vi "Flatten Value.vi"(8 "Error In":errorcluster, 11 "2D Path In":refnum<class "2D Path.lvclass">) -> (0 "Error Out":errorcluster, 1 "Value":string, 3 "2D Path Out":refnum<class "2D Path.lvclass">)   [LabVIEW 2017, in "Tree API.lvlib" / "2D Path.lvclass"]
doc: "Dynamic dispatch interface for flattening Tree Data classes to string."
uses:
  2D Path.lvclass
  Tree Manager/Tree.lvclass
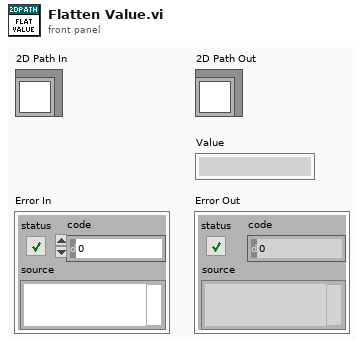
[diagram p1: front panel]
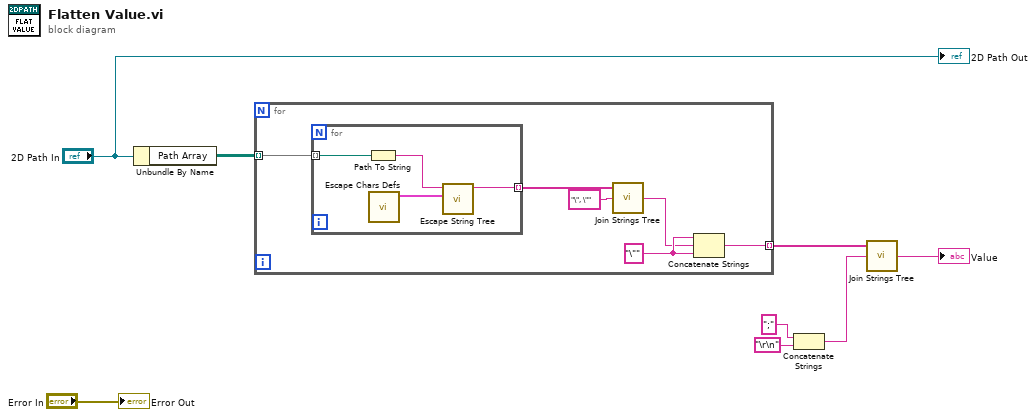
[diagram p0: block diagram]
diagram:
  n1 = Unbundle By Name("2D Path In") -> ("Path Array"=w8:path[][])
  n2 = for {
    tunnel: w8 -> [w14] mode=indexing
    tunnel: [w9] -> w6 mode=indexing
    w12 = "\"" ("string")
    n3 = for {
      tunnel: w14 -> [w18] mode=indexing
      tunnel: [w15] -> w10 mode=indexing
      n4 = Path To String(path=w18) -> (string=w16:string)
      n5 = call "Escape Chars Defs.vi"() -> ("Escapes"=w17:cluster{"String":string, "Escape":string}[])  [unwired: 11 in]
      n6 = call "Escape String Tree.vi"("Escapes"=w17, "String In"=w16) -> ("String Out"=w15:string)  [unwired: 9 in]
    }
    n7 = call "Join Strings Tree.vi"("Separator (,)"="\", \"", "Strings In"=w10) -> ("String"=w11:string)  [unwired: 1 in]
    n8 = Concatenate Strings(w12, w11, w12) -> (w9:string)
  }
  n9 = Concatenate Strings(";" ("Separator (,)"), "\r\n") -> (w3:string)
  n10 = call "Join Strings Tree.vi"("Separator (,)"=w3, "Strings In"=w6) -> ("String"=→"Value":string)  [unwired: 1 in]
  "2D Path Out" <- "2D Path In"
  "Error Out" <- "Error In"
